vi "LC-MISDK_Meas.vi"() -> ()   [LabVIEW 2015]
uses:
  C:/Users/e09031/Documents/GMA/LC-160/Labview/Sample_LC-MISDK/LC-MISDK.dll
  LC-MISDK.dll
panel:
  out "X":dbl
  out "Y":dbl
  out "Z":dbl
  out "Lv":dbl
  out "Dw":dbl
  out "Pe":dbl
  out "Lv":dbl
  out "Tcp":dbl
  out "Duv":dbl
  out "ReadLatestData Error":dbl format="%#_6f"
  out "Lv":dbl
  out "ud":dbl
  out "vd":dbl
  in  "Get Measurement Data":T1(radio)=enum."Lvxy"
  in  "Measurement":bool
  out "y":dbl
  out "x":dbl
  out "Lv":dbl
  out "Connect error Code":dbl
  in  "EXIT":bool
  in  "Connect":bool
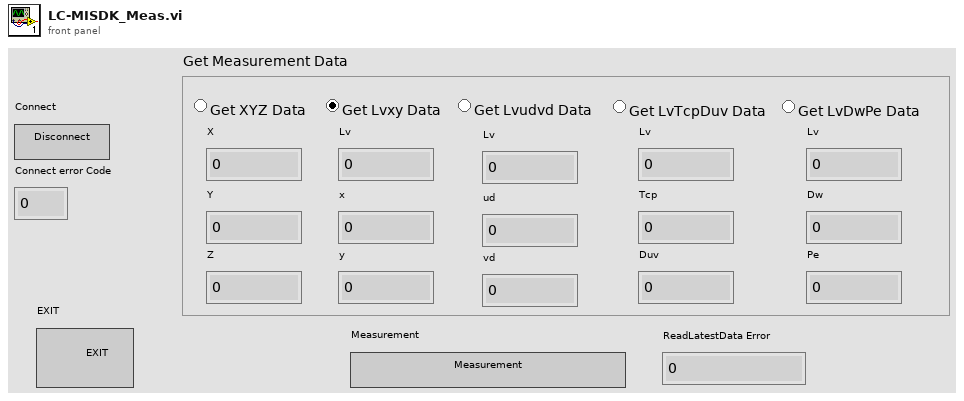
[diagram p1: front panel]
types:
  T1 = enum32{"XYZ", "Lvxy", "Lvudvd", "LvTcpDuv", "LvDwPe"}
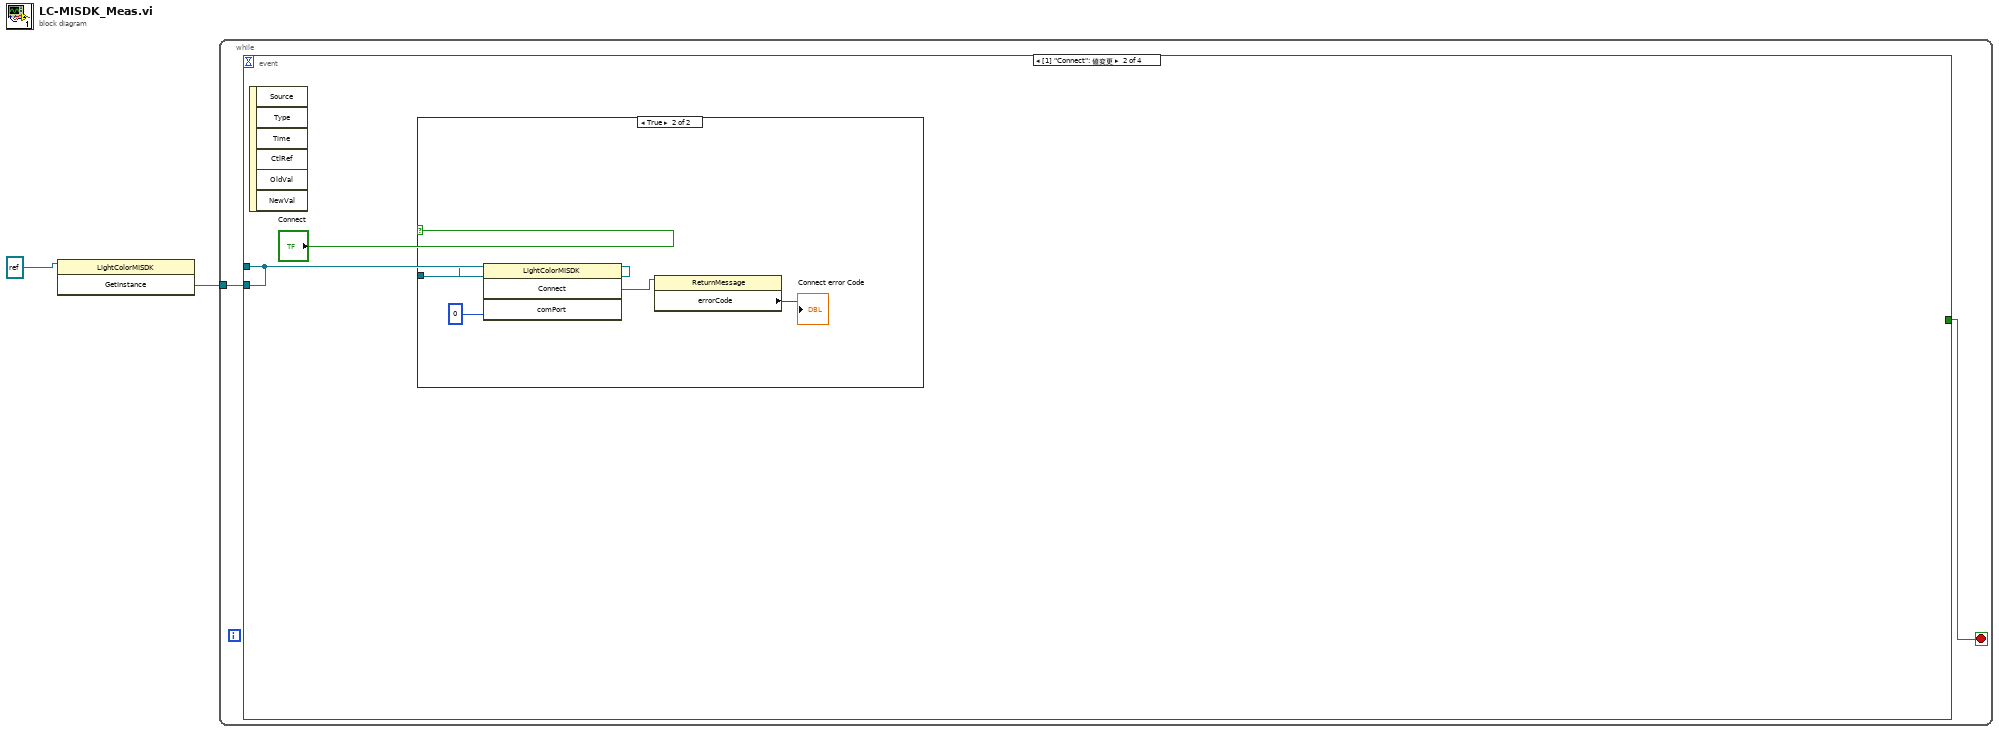
[diagram p0: block diagram]
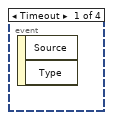
[diagram p2: hidden frame]
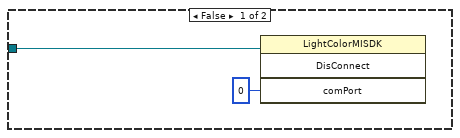
[diagram p3: hidden frame]
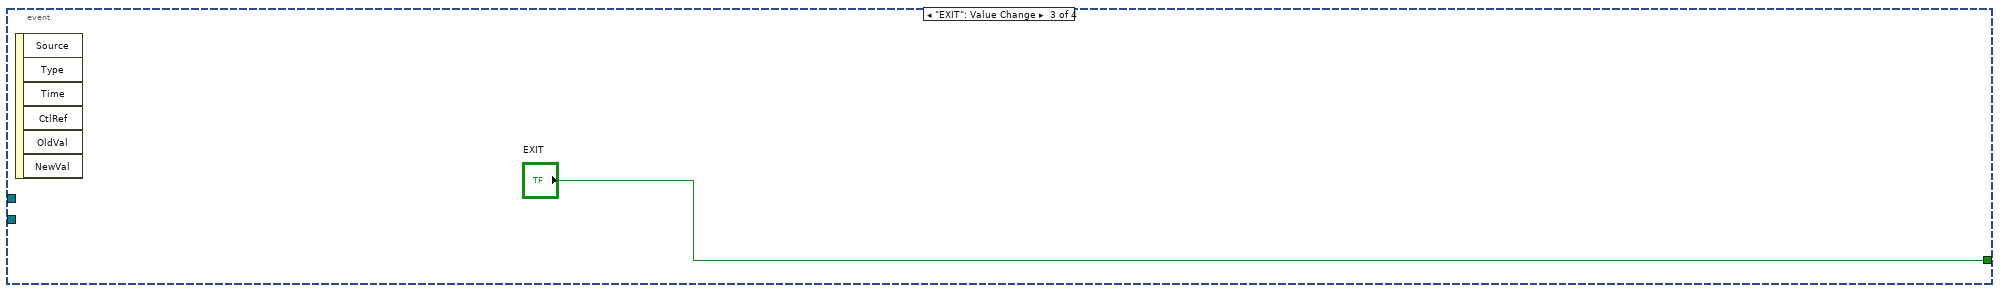
[diagram p4: hidden frame]
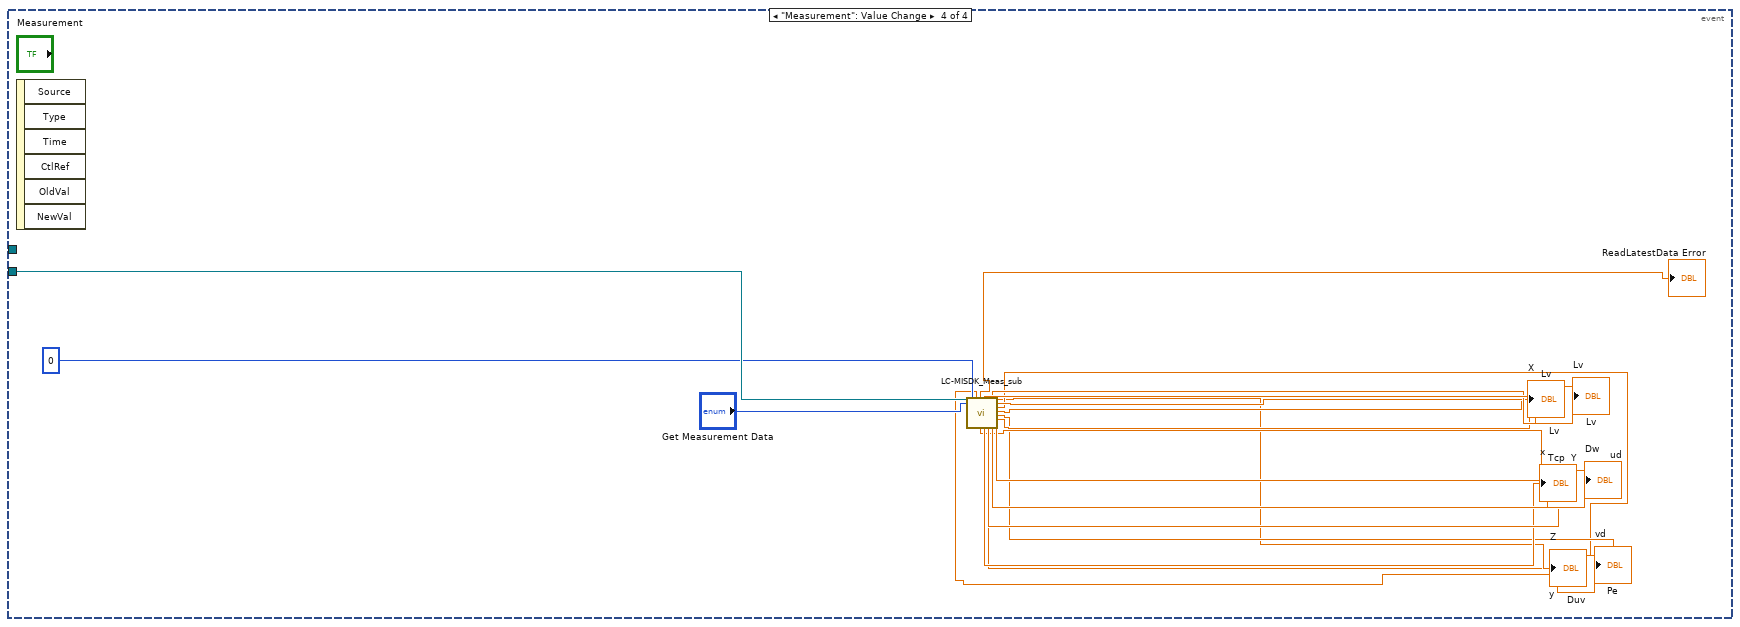
[diagram p5: hidden frame]
diagram:
  n1 = invoke on="インボークノード" class="LightColorMISDK" method="GetInstance"(reference=refnum<k24> refnum ("リファレンス出力")) -> ("GetInstance"=w1:refnum<k24>)  [unwired: 2 in, 2 out]
  n2 = while {
    tunnel: w1 -> [w4]
    stop <- w3 stop-if-true
    n3 = event shown="[1] \"Connect\": 値変更" {
      selector: _ -> [_ _ _ _]
      dyn-events: _ -> [_ _ _ _]
      timeout: _ -> [_ _ _ _]
      tunnel: [_ w5 _ _] -> _
      tunnel: [_ _ "EXIT" _] -> w3
      tunnel: w4 -> [_ w5 _ w32]
      event Timeout {
        n4 = event-data() -> ()  [unwired: 1 in, 2 out]
      }
      event "Connect": Value Change {
        n5 = event-data() -> ()  [unwired: 1 in, 6 out]
        n6 = case shown="TRUE" "Connect" {
          tunnel: w5 -> [w7 w12]
          frame False {
            n7 = invoke on="インボークノード" class="LightColorMISDK" method="DisConnect"(reference=w7, "comPort"=0) -> ()  [unwired: 2 in, 4 out]
          }
          frame True {
            n8 = invoke on="インボークノード" class="LightColorMISDK" method="Connect"(reference=w12, "comPort"=0) -> ("Connect"=w9:refnum<k24>)  [unwired: 2 in, 3 out]
            n9 = property on="プロパティノード" class="ReturnMessage"(reference=w9) -> ("errorCode"=→"Connect error Code":i32)  [unwired: 1 in, 2 out]
          }
        }
      }
      event "EXIT": Value Change {
        n10 = event-data() -> ()  [unwired: 1 in, 6 out]
      }
      event "Measurement": Value Change {
        n11 = event-data() -> ()  [unwired: 1 in, 6 out]
        n12 = call "LC-MISDK_Meas_sub.vi"(".NET refnum入力"=w32, "Get Measurement Data"="Get Measurement Data", "数値"=0) -> ("Duv"=→"Duv":dbl, "ReadLatestData Error"=→"ReadLatestData Error":dbl, "Tcp"=→"Tcp":dbl, "Lv 4"=→"Lv":dbl, "x"=→"x":dbl, "Z"=→"Z":dbl, "Y"=→"Y":dbl, "Lv 3"=→"Lv":dbl, "Dw"=→"Dw":dbl, "y"=→"y":dbl, "Lv"=→"Lv":dbl, "Pe"=→"Pe":dbl, "X"=→"X":dbl, "vd"=→"vd":dbl, "Lv 2"=→"Lv":dbl, "ud"=→"ud":dbl)  [unwired: 9 in]
      }
    }
  }
